vi "Reference_Data_Read.vi"(6 "Active Sensors":bool[](array[boolean]), 7 "chkeach_ch":bool, 8 "error in":errorcluster caption="错误输入", 9 "ILSTS":refnum<k24>, 10 "Data_struct":refnum<k24>[](array[refnum]), 11 "TSL":refnum<k24>) -> (0 "error IO":errorcluster)   [LabVIEW 2017]
doc: "// Reference Data Read\n// This function must use after \"SET\""
uses:
  D:/test/ILSTS/LV_IL/LV_IL_Sample_x64/DLL/STSProcess.dll
  DLL/STSProcess.dll
  D:/test/ILSTS/LV_IL/LV_IL_Sample_x64/DLL/InstrumentDLL.dll
  DLL/InstrumentDLL.dll
  <vilib>/Utility/file.llb/Read Delimited Spreadsheet (string).vi
panel:
  in  "txtstepwave":dbl caption="WavelengthStep(nm)"
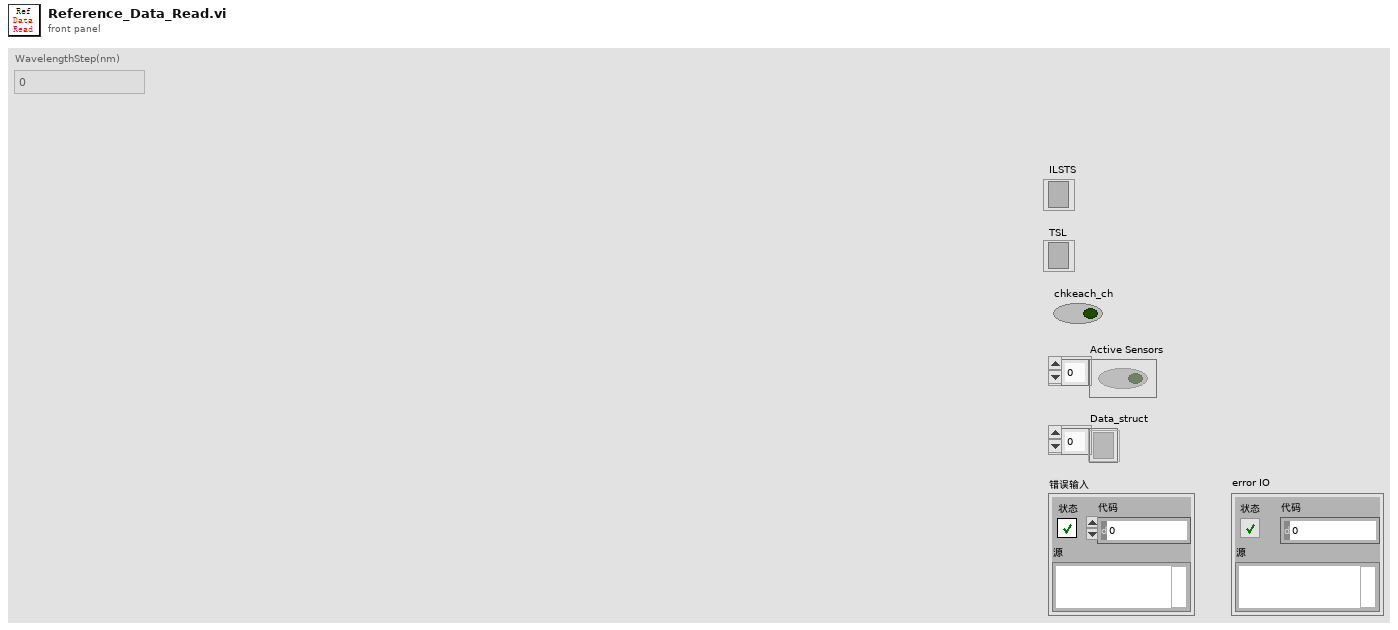
[diagram p1: front panel]
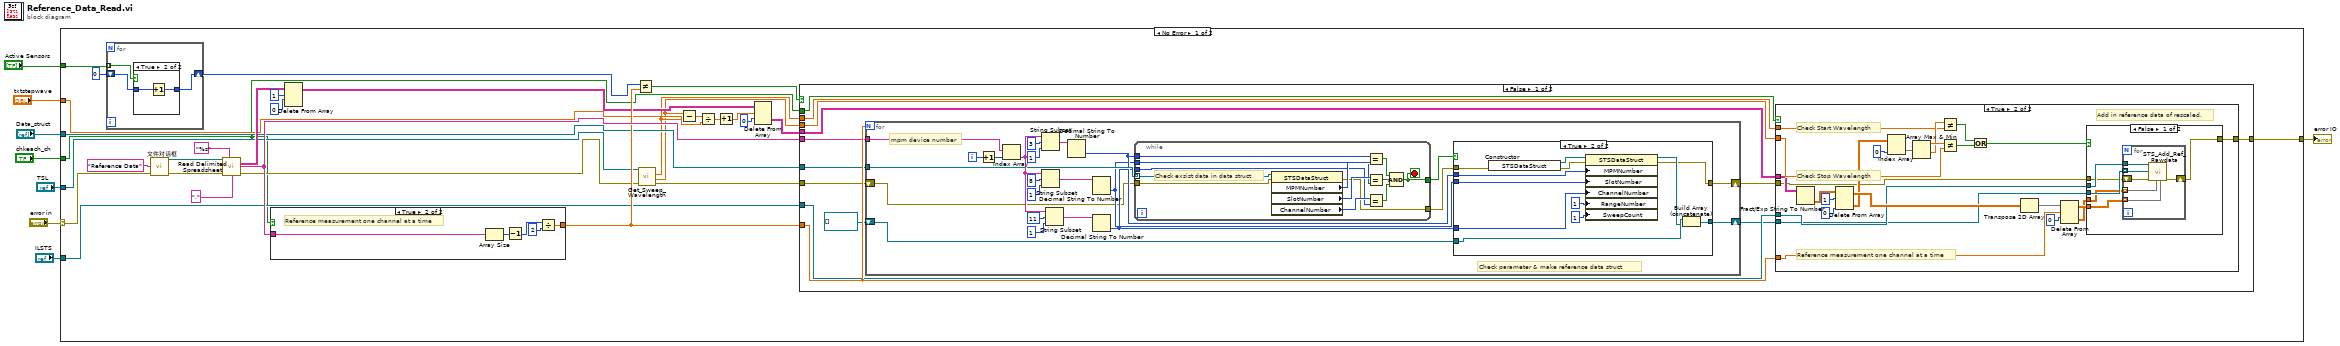
[diagram p0: block diagram]
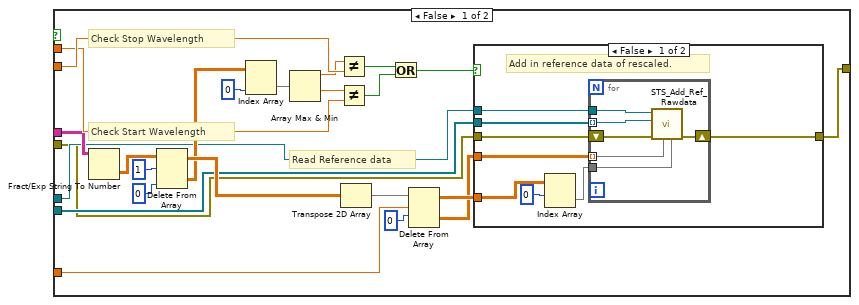
[diagram p2: hidden frame]
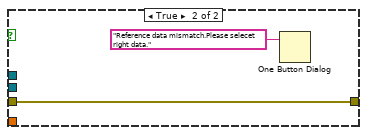
[diagram p3: hidden frame]
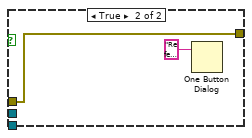
[diagram p4: hidden frame]
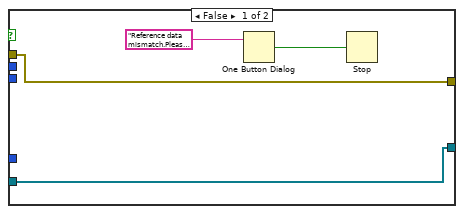
[diagram p5: hidden frame]
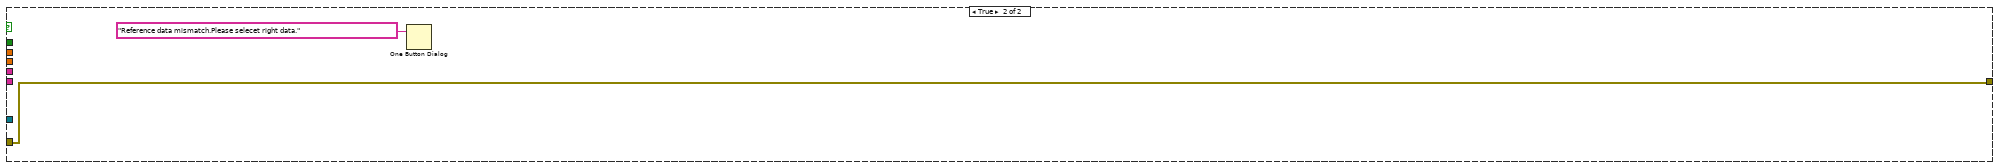
[diagram p6: hidden frame]
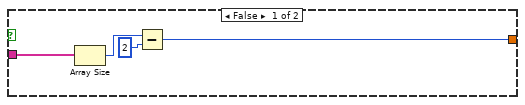
[diagram p8: hidden frame]
diagram:
  n1 = case shown="No Error" "error in" {
    selector: "error in" -> [w25 w200]
    tunnel: "ILSTS" -> [w32 _]
    tunnel: [w24 w200] -> w6
    tunnel: "Data_struct" -> [w22 _]
    tunnel: "TSL" -> [w21 _]
    tunnel: "Active Sensors" -> [w20 _]
    tunnel: "txtstepwave" -> [w19 _]
    tunnel: "chkeach_ch" -> [w18 _]
    frame No Error {
      n2 = for {
        shift-right: [w186] -> w36
        shift-left: 0 -> [w187]
        tunnel: w20 -> [w185] mode=indexing
        n3 = case shown="True" w185 {
          tunnel: w187 -> [w188 w190]
          tunnel: [w188 w189] -> w186
          frame False {
          }
          frame True {
            n4 = Increment(x=w190) -> (x+1=w189:i32)
          }
        }
      }
      n5 = call "文件对话框"("default name"="Reference Data", "error in"=w25) -> ("selected path"=w37:path, "error out"=w38:errorcluster)  [unwired: 10 in, 2 out]
      n6 = call-poly <vilib>:"Read Delimited Spreadsheet.vi"("file path (dialog if empty)"=w37, "format (%s)"="%s", "error in (no error)"=w38, "delimiter (\\t)"="," ("delimiter (\\t)")) -> ("all rows"=w27:string[][], "first row"=w39:string[], "error out"=w23:errorcluster)  [unwired: 6 in, 3 out]
      n7 = case shown="True" w18 {
        tunnel: w39 -> [w194 w199]
        tunnel: [w192 w196] -> w33
        frame False {
          n8 = Array Size(array=w194) -> (size(s)=w191:i32)
          n9 = Subtract(x=w191, y=2) -> (x-y=w192:i32)
        }
        frame True {
          # "Reference measurement one channel at a time"
          n10 = Array Size(array=w199) -> (size(s)=w195:i32)
          n11 = Decrement(x=w195) -> (x-1=w198:i32)
          n12 = Divide(x=w198, y=2) -> (x/y=w196:dbl)
        }
      }
      n13 = Delete From Array(array=w27, length=1 ("长度"), index (row)=0 ("索引 (行)")) -> (array with subset deleted=w26:string[][])  [unwired: 1 in, 1 out]
      n14 = Not Equal?(x=w36, y=w33) -> (x != y?=w17:bool)
      n15 = call "Get_Sweep_Wavelength.vi"("error in (no error)"=w23, ".NET Reference in"=w21) -> ("error out"=w9:errorcluster, "endwave out"=w10:dbl, "startwave out"=w11:dbl)  [unwired: 6 in, 1 out]
      n16 = Subtract(x=w10, y=w11) -> (x-y=w16:dbl)
      n17 = Divide(x=w16, y=w19) -> (x/y=w15:dbl)
      n18 = Increment(x=w15) -> (x+1=w14:dbl)
      n19 = Delete From Array(array=w26, length=w14, index (row)=0 ("索引 (行)")) -> (deleted portion=w12:string[][])  [unwired: 1 in, 1 out]
      n20 = case shown="False" w17 {
        tunnel: w33 -> [w52 _]
        tunnel: w39 -> [w51 _]
        tunnel: w22 -> [w50 _]
        tunnel: w18 -> [w49 _]
        tunnel: w12 -> [w48 _]
        tunnel: w10 -> [w47 _]
        tunnel: w32 -> [w44 _]
        tunnel: w11 -> [w46 _]
        tunnel: [w42 w183] -> w24
        tunnel: w9 -> [w41 w183]
        frame False {
          n21 = for {
            N: w52 -> [_]
            tunnel: w51 -> [w153]
            tunnel: w50 -> [w143]
            shift-right: [w135] -> w43
            shift-left: refnum<k24>[] [] ("Data_struct") -> [w134]
            shift-right: [w131] -> w40
            shift-left: w41 -> [w133]
            i -> [w148]
            # "Check parameter & make reference data struct"
            # "mpm device number"
            n22 = Increment(x=w148) -> (x+1=w147:i32)
            n23 = Index Array(array=w153, index=w147) -> (element=w144:string)
            n24 = String Subset(string=w144, offset (0)=3 ("偏移量(0)"), length (rest)=1 ("长度（剩余）")) -> (substring=w140:string)
            n25 = String Subset(string=w144, offset (0)=8 ("偏移量(0)"), length (rest)=1 ("长度（剩余）")) -> (substring=w139:string)
            n26 = String Subset(string=w144, offset (0)=11 ("偏移量(0)"), length (rest)=1 ("长度（剩余）")) -> (substring=w141:string)
            n27 = Decimal String To Number(string=w140) -> (number=w138:i32)  [unwired: 2 in, 1 out]
            n28 = Decimal String To Number(string=w139) -> (number=w137:i32)  [unwired: 2 in, 1 out]
            n29 = Decimal String To Number(string=w141) -> (number=w136:i32)  [unwired: 2 in, 1 out]
            n30 = while {
              tunnel: w143 -> [w166] mode=indexing
              tunnel: [w159] -> w142
              tunnel: w136 -> [w158]
              tunnel: w138 -> [w157]
              tunnel: w137 -> [w156]
              tunnel: w133 -> [w155]
              tunnel: [w154] -> w132
              stop <- w159 stop-if-true
              # "Check exsist data in data struct"
              n31 = property on="属性节点" class="STSDataStruct"(reference=w166, error in=w155) -> (error out=w154:errorcluster, "MPMNumber"=w165:i32, "SlotNumber"=w164:i32, "ChannelNumber"=w163:i32)  [unwired: 1 out]
              n32 = Equal?(x=w157, y=w165) -> (x = y?=w162:bool)
              n33 = Equal?(x=w164, y=w156) -> (x = y?=w161:bool)
              n34 = Equal?(x=w163, y=w158) -> (x = y?=w160:bool)
              n35 = Compound Arithmetic op=AND ("复合运算")(w162, w161, w160) -> (w159:bool)
            }
            n36 = case shown="True" w142 {
              tunnel: w138 -> [_ w182]
              tunnel: w137 -> [_ w181]
              tunnel: w136 -> [_ w180]
              tunnel: w134 -> [w169 w177]
              tunnel: [w169 w175] -> w135
              tunnel: w132 -> [w167 w172]
              tunnel: [w167 w171] -> w131
              frame False {
                n37 = One Button Dialog(message="Reference data mismatch.Please selecet right data." ("消息")) -> (true=w168:bool)  [unwired: 1 in]
                n38 = Stop(stop? (T)=w168) -> ()
              }
              frame True {
                n39 = constructor class="STSDataStruct"(error in=w172) -> (reference out=w174:refnum<k24>, error out=w173:errorcluster)  [unwired: 2 in, 1 out]
                n40 = property on="属性节点" class="STSDataStruct"(reference=w174, error in=w173, "MPMNumber"=w182, "SlotNumber"=w181, "ChannelNumber"=w180, "RangeNumber"=1, "SweepCount"=1) -> (reference out=w176:refnum<k24>, error out=w171:errorcluster)
                n41 = Build Array (concatenate)(w177, w176) -> (w175:refnum<k24>[])
              }
            }
          }
          n42 = case shown="True" w49 {
            tunnel: w48 -> [w62 w102]
            tunnel: w52 -> [w65 w105]
            tunnel: w47 -> [w76 w116]
            tunnel: w46 -> [w63 w103]
            tunnel: w43 -> [w58 w95]
            tunnel: w44 -> [w55 w98]
            tunnel: [w54 w93] -> w42
            tunnel: w40 -> [w53 w94]
            frame False {
              # "Check Stop Wavelength"
              # "Check Start Wavelength"
              # "Read Reference data"
              n43 = Fract/Exp String To Number(string=w62) -> (number=w75:dbl[][])  [unwired: 3 in, 1 out]
              n44 = Delete From Array(array=w75, length=1 ("长度"), index (col)=0 ("禁用的索引 (列)")) -> (deleted portion=w71:dbl[][], array with subset deleted=w72:dbl[][])  [unwired: 1 in]
              n45 = Index Array(array=w71, index (col)=0 ("禁用的索引 (列)")) -> (element=w69:dbl[])  [unwired: 1 in]
              n46 = Array Max & Min(array=w69) -> (max value=w68:dbl, min value=w67:dbl)  [unwired: 2 out]
              n47 = Not Equal?(x=w68, y=w76) -> (x != y?=w61:bool)
              n48 = Not Equal?(x=w67, y=w63) -> (x != y?=w60:bool)
              n49 = Transpose 2D Array(2D array=w72) -> (transposed array=w66:dbl[][])
              n50 = Or(x=w61, y=w60) -> (x .or. y?=w59:bool)
              n51 = Delete From Array(array=w66, length=w65, index (row)=0 ("索引 (行)")) -> (deleted portion=w56:dbl[][], array with subset deleted=w57:dbl[][])  [unwired: 1 in]
              n52 = case shown="False" w59 {
                tunnel: w55 -> [w84 _]
                tunnel: w58 -> [w83 _]
                tunnel: w57 -> [w81 _]
                tunnel: w56 -> [w82 _]
                tunnel: [w78 w91] -> w54
                tunnel: w53 -> [w77 w91]
                frame False {
                  # "Add in reference data of rescaled."
                  n53 = Index Array(array=w81, index (row)=0 ("索引 (行)")) -> (element=w79:dbl[])  [unwired: 1 in]
                  n54 = for {
                    tunnel: w84 -> [w90]
                    tunnel: w83 -> [w89] mode=indexing
                    tunnel: w82 -> [w88] mode=indexing
                    tunnel: w79 -> [w87]
                    shift-right: [w86] -> w78
                    shift-left: w77 -> [w85]
                    n55 = call "STS_Add_Ref_Rawdata.vi"("monitorData"=w87, "MPMData"=w88, "错误输入（无错误）"=w85, "Setting"=w89, "STSProcess.ILSTS"=w90) -> ("错误输出"=w86:errorcluster)  [unwired: 5 in, 1 out]
                  }
                }
                frame True {
                  n56 = One Button Dialog(message="Reference data mismatch.Please selecet right data." ("消息")) -> ()  [unwired: 1 in, 1 out]
                }
              }
            }
            frame True {
              # "Add in reference data of rescaled."
              # "Check Stop Wavelength"
              # "Check Start Wavelength"
              # "Reference measurement one channel at a time"
              n57 = Fract/Exp String To Number(string=w102) -> (number=w115:dbl[][])  [unwired: 3 in, 1 out]
              n58 = Delete From Array(array=w115, length=1 ("长度"), index (col)=0 ("禁用的索引 (列)")) -> (deleted portion=w111:dbl[][], array with subset deleted=w112:dbl[][])  [unwired: 1 in]
              n59 = Index Array(array=w111, index (col)=0 ("禁用的索引 (列)")) -> (element=w109:dbl[])  [unwired: 1 in]
              n60 = Array Max & Min(array=w109) -> (max value=w108:dbl, min value=w107:dbl)  [unwired: 2 out]
              n61 = Not Equal?(x=w107, y=w103) -> (x != y?=w100:bool)
              n62 = Not Equal?(x=w108, y=w116) -> (x != y?=w101:bool)
              n63 = Or(x=w100, y=w101) -> (x .or. y?=w99:bool)
              n64 = Transpose 2D Array(2D array=w112) -> (transposed array=w106:dbl[][])
              n65 = Delete From Array(array=w106, length=w105, index (row)=0 ("索引 (行)")) -> (deleted portion=w96:dbl[][], array with subset deleted=w97:dbl[][])  [unwired: 1 in]
              n66 = case shown="False" w99 {
                tunnel: w98 -> [w122 _]
                tunnel: w95 -> [w121 _]
                tunnel: w97 -> [w120 _]
                tunnel: w96 -> [w119 _]
                tunnel: w94 -> [w118 w129]
                tunnel: [w117 w129] -> w93
                frame False {
                  n67 = for {
                    tunnel: w122 -> [w128]
                    tunnel: w121 -> [w127] mode=indexing
                    tunnel: w120 -> [w126] mode=indexing
                    tunnel: w119 -> [w125] mode=indexing
                    shift-right: [w123] -> w117
                    shift-left: w118 -> [w124]
                    n68 = call "STS_Add_Ref_Rawdata.vi"("monitorData"=w126, "MPMData"=w125, "错误输入（无错误）"=w124, "Setting"=w127, "STSProcess.ILSTS"=w128) -> ("错误输出"=w123:errorcluster)  [unwired: 5 in, 1 out]
                  }
                }
                frame True {
                  n69 = One Button Dialog(message="Reference data mismatch.Please selecet right data." ("消息")) -> ()  [unwired: 1 in, 1 out]
                }
              }
            }
          }
        }
        frame True {
          n70 = One Button Dialog(message="Reference data mismatch.Please selecet right data." ("消息")) -> ()  [unwired: 1 in, 1 out]
        }
      }
    }
    frame Error {
    }
  }
  "error IO" <- w6
